vi "Create.vi"(8 "Error In":errorcluster, 11 "reference in":refnum<class "Communicator.lvclass">) -> (0 "Error Out":errorcluster, 3 "reference out":refnum<class "Communicator.lvclass">)   [LabVIEW 2024, in "Communicator.lvclass"]
uses:
  Communicator.lvclass
  Communicator.lvclass/Communicator.ctl
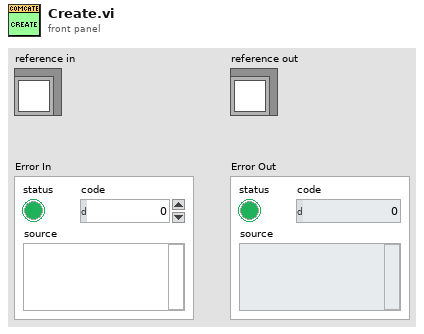
[diagram p1: front panel]
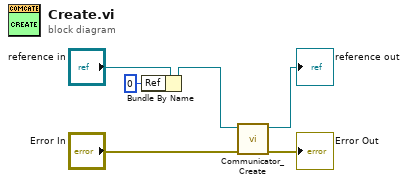
[diagram p0: block diagram]
diagram:
  n1 = Bundle By Name(cluster="reference in", "Ref"=u32 0) -> (w4:refnum<class "Communicator.lvclass">)
  n2 = call "Communicator_Create.vi"("Error In"="Error In", "Communicator in"=w4) -> ("Error Out"=→"Error Out":errorcluster, "Communicator out"=→"reference out":refnum<class "Communicator.lvclass">)  [unwired: 8 in]
